vi "tes assemble (fuzzy).vi"() -> ()   [LabVIEW 2015]
uses:
  <vilib>/userdefined/High Color/IMAQdx.ctl
  <vilib>/Platform/TimedLoop/XDataNode/timing_clust.ctl
  <vilib>/Platform/TimedLoop/XDataNode/nitl_modes.ctl
  <vilib>/Platform/TimedLoop/XDataNode/wakeup.ctl
  <vilib>/FPGAPlugInAG/myRIO-1900/niLvFpga_Open_myRIO-1900.vi
  <vilib>/rvi/interface/common/dynamic/niFpgaDynamicAddResources.vi
  <vilib>/FPGAPlugInAG/Dynamic/niLvFpga_Run_Dynamic.vi
  <vilib>/Utility/error.llb/Error Cluster From Error Code.vi
  <vilib>/rvi/errors/niLvFpgaAdjustHostInterfaceError.vi
  <vilib>/FPGAPlugInAG/Dynamic/niLvFpga_Close_Dynamic.vi
  <vilib>/addons/control/pid/pid.llb/PID (DBL).vi
  <vilib>/addons/Fuzzy Logic/FL Fuzzy Controller (MIMO).vi
  <vilib>/Platform/TimedLoop/XDataNode/XDataNode.xnode
  <vilib>/rvi/interface/nirviOpenFPGA/nirviOpenFPGA.xnode
  TA/FPGA Bitfiles/FPGAv2_FPGATarget2_Assemble_19Xc0cZodWc.lvbitx
  Assemble.vi
  <vilib>/rvi/interface/nirviMethod/nirviMethod.xnode
  <vilib>/rvi/interface/nirviReadWriteControl/nirviReadWriteControl.xnode
  <vilib>/rvi/interface/nirviCloseFPGA/nirviCloseFPGA.xnode
  <vilib>/rvi/interface/Simulation/niFpgaSimulationCallBeginRW.vi
  <vilib>/Platform/TimedLoop/XDataNode/XDNodeRunTimeDep.lvlib
  <vilib>/vision/driver/NI_Vision_Acquisition_Software.lvlib
  <resource>/objmgr/imaqdx.rc
  <vilib>/addons/control/pid/NI_PID_pid.lvlib
  NiFpgaLv.dll
  <vilib>/addons/Fuzzy Logic/NI_Fuzzy_Logic_API.lvlib
panel:
  out "voltage":dbl
  out "var.RTH":dbl
  out "kec.kanan":dbl
  out "kec.kiri":dbl
  out "kecp.kanan":dbl
  out "kecp.kiri":dbl
  out "var.auto":dbl
  out "Return to Home":dbl
  out "s 4":dbl
  out "s 3":dbl
  out "s 2":dbl
  out "s1":dbl
  out "var. auto":dbl
  in  "Mode":bool
  in  "Run/Stop":bool
  in  "RTH":bool
  in  "Enc1 Reset":bool
  in  "Enc2 Reset":bool
  in  "Enc3 Reset":bool
  in  "Enc4 Reset":bool
  in  "Tfu":u32=10
  out "lf 2":dbl
  out "fr 2":i32
  out "fw 2":i32
  out "fl 2":i32
  out "br 2":dbl
  out "bw 2":i32
  out "rg 2":dbl
  out "st 2":i32
  in  "Trigger pulse interval  4":u32
  in  "Trigger pulse interval  3":u32
  in  "Trigger pulse interval  2":u32
  in  "Trigger pulse interval 1":u32
  out "Motor Response-Set Point vs. AcualSpeed":cluster{dbl, "Velocity (Counts/Interval)":i32}(graph)
  out "relay 4":bool
  out "relay 3":bool
  out "relay 2":bool
  out "relay1":bool
  out "bocor 2":bool
  out "Water_LVL2":u16
  out "Water_LVL1":u16
  out "bocor 1":bool
  out "Arus 4":dbl
  out "Arus 3":dbl
  out "Arus 2":dbl
  out "Arus1":dbl
  out "En 8":bool
  out "En 7":bool
  out "En 6":bool
  out "En 5":bool
  out "En 4":bool
  out "En 3":bool
  out "En 2":bool
  out "En 1":bool
  out "Rpm 4":i32
  out "Rpm 3":i32
  out "Rpm 2":i32
  out "Rpm 1":i32
  out "To":u32
  out "var. manual":dbl
  out "enc 4":i32
  out "enc 3":i32
  out "enc 2":i32
  out "enc 1":i32
  out "Time On4":dbl format="%.2f"
  out "Time On3":dbl format="%.2f"
  out "Time On2":dbl
  out "y position":dbl
  out "x position":dbl
  out "angle":dbl
  out "jarak tempuh":dbl
  out "Tf":u32
  out "Time On1":dbl
  out "distance4":sgl
  out "distance3":sgl
  out "distance2":sgl
  out "distance1":sgl
  out "Image":T1(plugin-control)
  in  "Image Type":T2 items=["Grayscale (U8)", "Grayscale (I16)", "Grayscale (SGL)", "Complex (CSG)", "RGB (U32)", "HSL (U32)", "RGB (U64)", "Grayscale (U16)"]
  in  "Border Size":i32=3
  in  "Session In":T3
  out "Channel 2":u32
  out "Channel 1":u32
  out "US 4":u32
  out "US3":u32
  out "US2":u32
  out "US1":u32
  out "STOP Indicator":bool
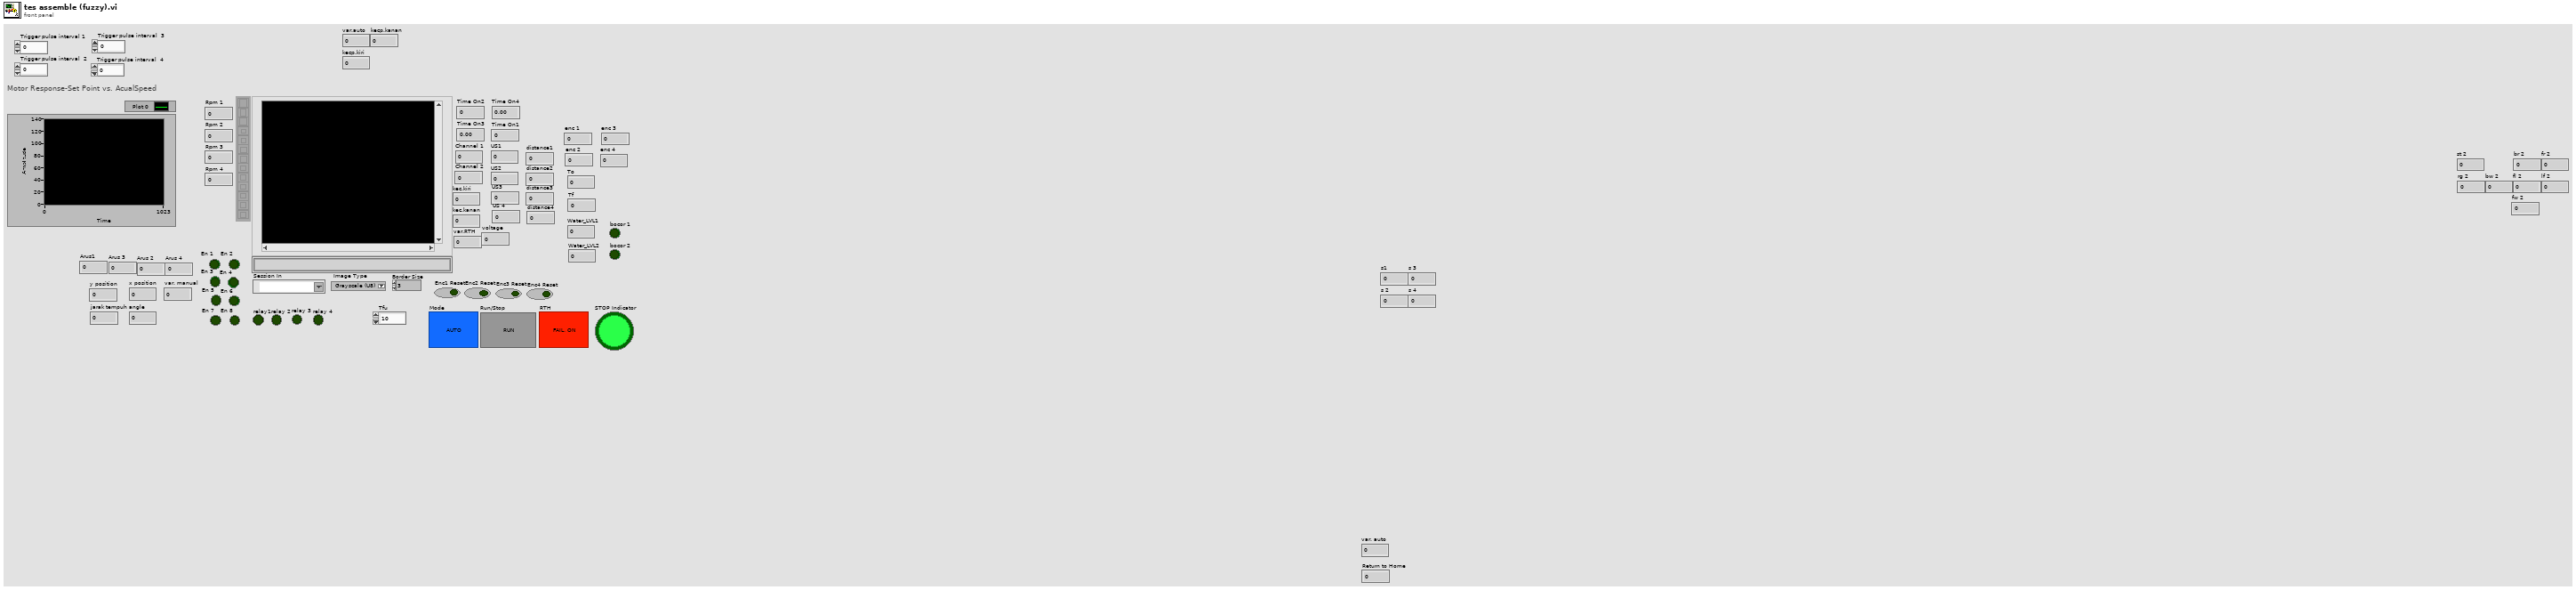
[diagram p1: front panel]
types:
  T1 = typedef "IMAQ Image.ctl" = refnum<image>
  T2 = typedef "Image Type" = u32
  T3 = typedef "IMAQdx.ctl" = refnum<k21>
  T4 = typedef "XDNodeRunTimeDep.lvlib/timing_clust.ctl" = cluster{"Expected End [f-1]":u64, "Actual End [f-1]":u64, "Finished Late? [f-1]":bool, "Expected End [i-1]":u64, "Actual End [i-1]":u64, "Finished Late? [i-1]":bool, "Expected Start [i]":u64, "Actual Start [i]":u64, "Expected Start [f]":u64, "Actual Start [f]":u64, "Source Name":string, "Structure Name":string, "Period":i64, "Deadline":i64, "Offset":i64, "Start":i64, "Priority":i32, "Timeout":i32, "Mode":T5, "Wakeup Reason":T6, "Error":errorcluster, "Source Type":string, "Secondary Source Type":string, "Global End Time":u64, "Global Start Time":u64, "Frame Duration":u64, "Iteration Duration":u64, "Assigned CPU":i32, "I/O Scan Engine Mode":u32}
  T5 = typedef "XDNodeRunTimeDep.lvlib/nitl_modes.ctl" = enum32{"No Change", "Process missed periods, maintain original phase", "Discard missed periods, maintain original phase", "Process missed periods, ignore original phase", "Discard missed periods, ignore original phase"}
  T6 = typedef "XDNodeRunTimeDep.lvlib/wakeup.ctl" = enum32{"Normal", "Aborted", "Asynchronous wakeup", "Timing source error", "Timed loop error", "Timeout"}
  T7 = cluster{"proportional gain (Kc)":dbl, "integral time (Ti, min)":dbl, "derivative time (Td, min)":dbl}
  T8 = typedef "NI_Fuzzy_Logic_API.lvlib/FL System.ctl" = cluster{"input variables":T9[], "output variables":T9[], "rules":T12[], "defuzzification method":T18, "description":string, "user MF interpolating polynomials":T19[]}
  T9 = typedef "NI_Fuzzy_Logic_API.lvlib/FL Variable.ctl" = cluster{"name":string, "range":dbl[], "MFs":T10[]}
  T10 = typedef "NI_Fuzzy_Logic_API.lvlib/FL Membership Function.ctl" = cluster{"name":string, "shape":T11, "points":dbl[], "color":u32, "user-defined shape index":i32}
  T11 = typedef "NI_Fuzzy_Logic_API.lvlib/FL Membership Function Shape.ctl" = u16
  T12 = typedef "NI_Fuzzy_Logic_API.lvlib/FL Rule.ctl" = cluster{"antecedents":T13[], "antecedent connective":T15, "consequents":T16[], "consequent implication":T17, "degree of support":dbl}
  T13 = typedef "NI_Fuzzy_Logic_API.lvlib/FL Antecedent.ctl" = cluster{"Var Index":i32, "MF Index":i32, "Cond":T14}
  T14 = typedef "NI_Fuzzy_Logic_API.lvlib/FL Modifier.ctl" = u16
  T15 = typedef "NI_Fuzzy_Logic_API.lvlib/FL Antecedent Connective.ctl" = u16
  T16 = typedef "NI_Fuzzy_Logic_API.lvlib/FL Consequent.ctl" = cluster{"Var Index":i32, "MF Index":i32, "Cond":T14}
  T17 = typedef "NI_Fuzzy_Logic_API.lvlib/FL Consequent Implication.ctl" = u16
  T18 = typedef "NI_Fuzzy_Logic_API.lvlib/FL Defuzzification.ctl" = u16
  T19 = typedef "NI_Fuzzy_Logic_API.lvlib/FL Interpolating polynomials.ctl" = cluster{"X":dbl[], "Y":dbl[], "Y(x) coeff":dbl[][], "X(y) coeff":dbl[][], "Area(y) coeff":dbl[][], "coa_x(y) coeff":dbl[][]}
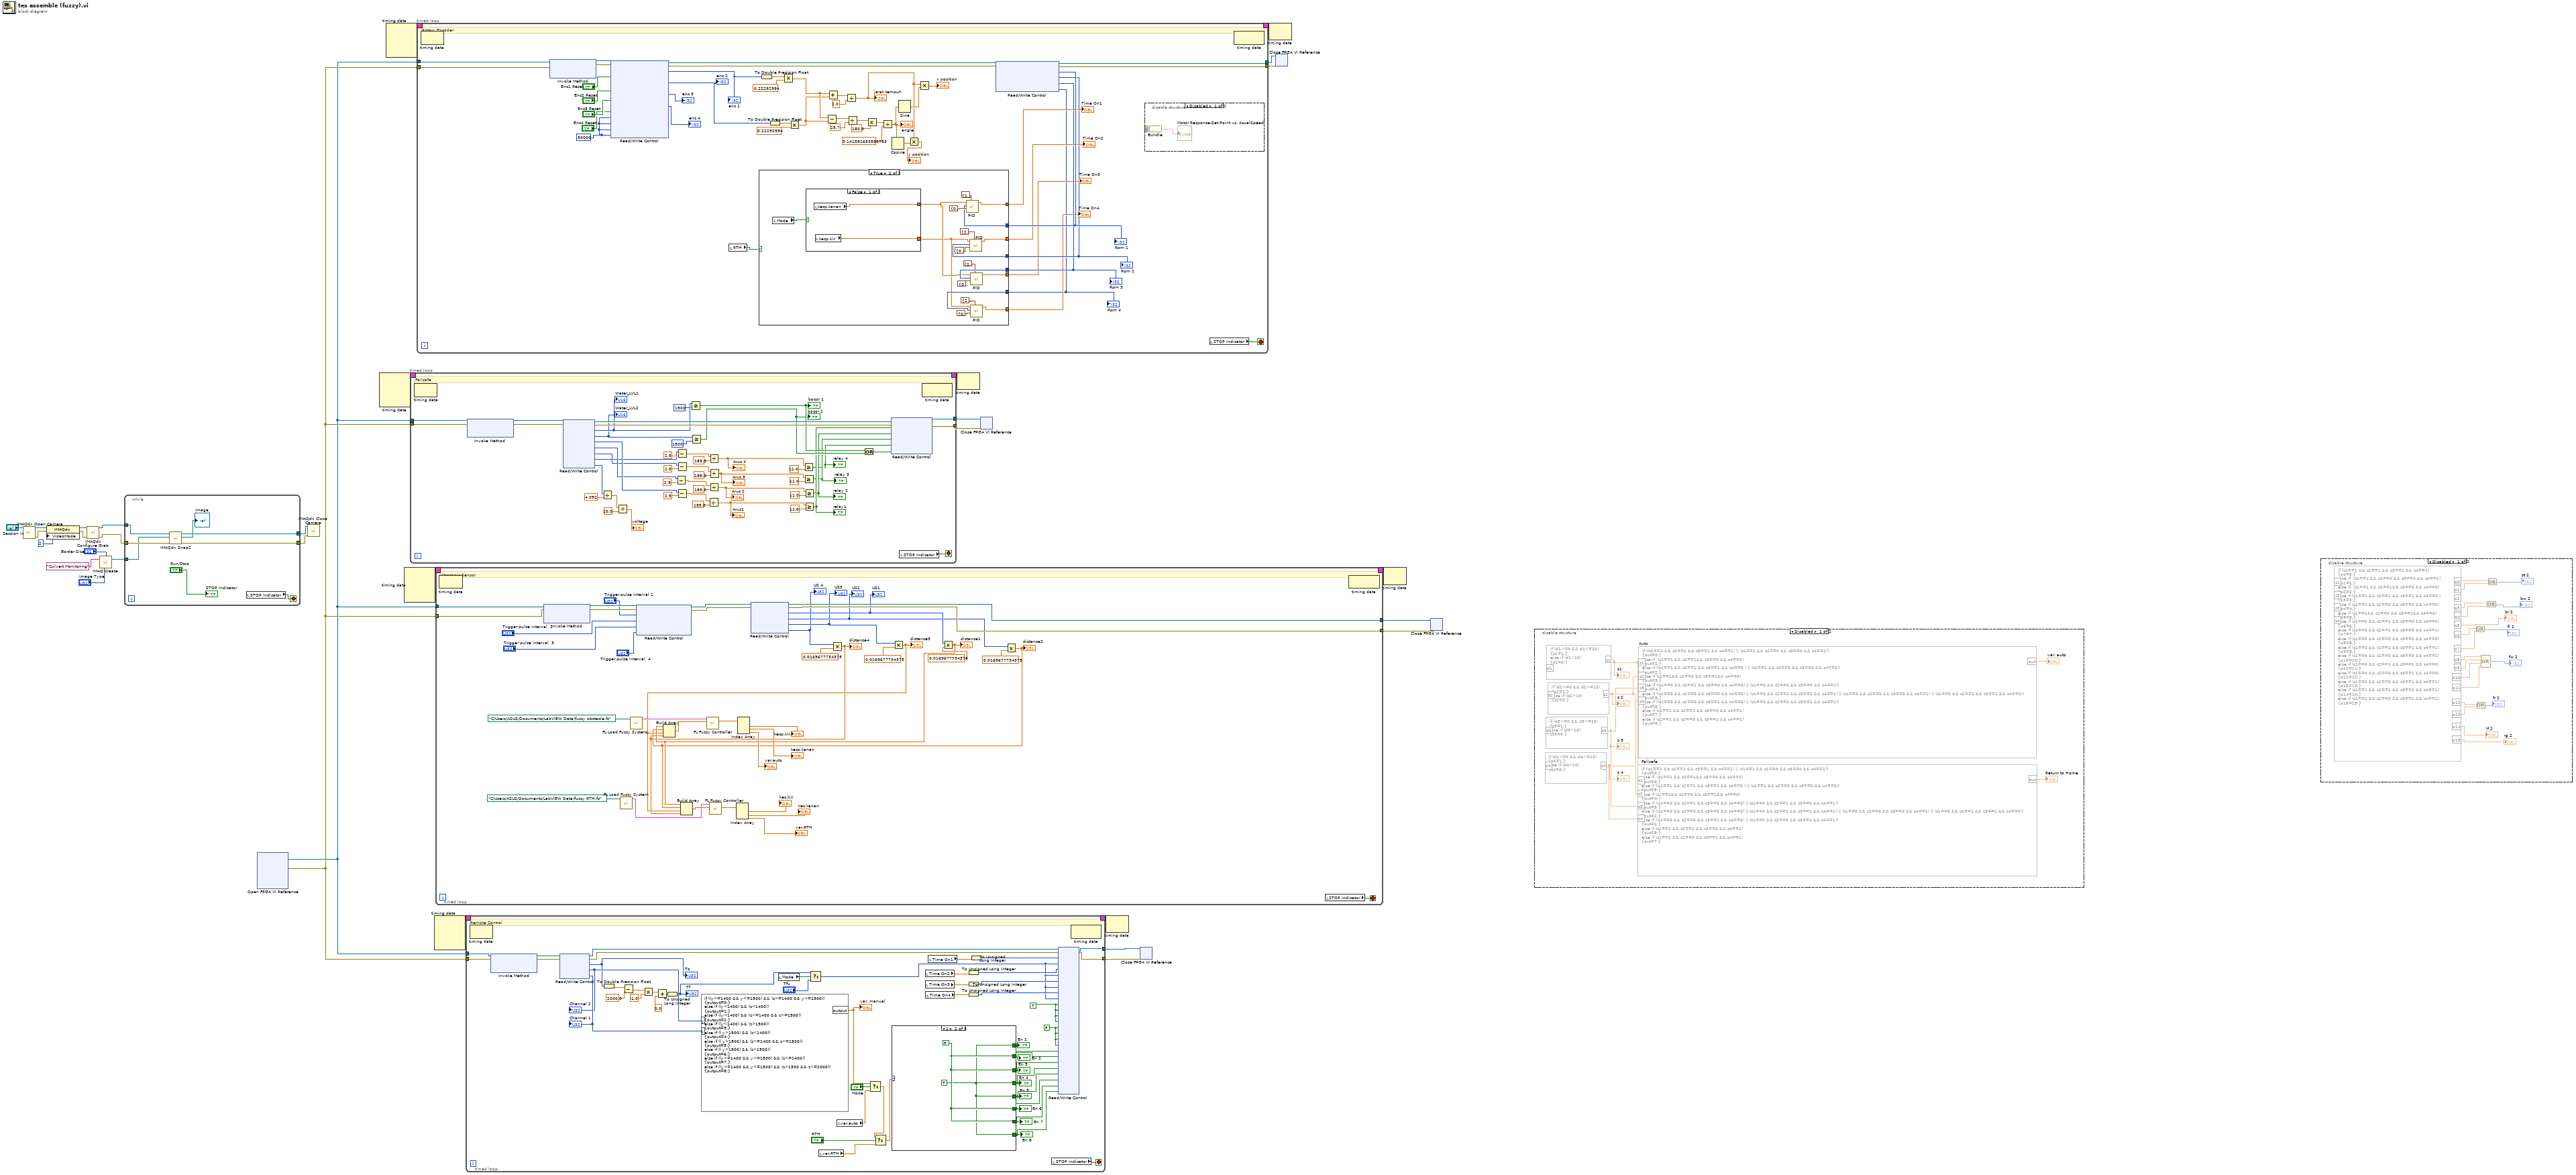
[diagram p0: block diagram]
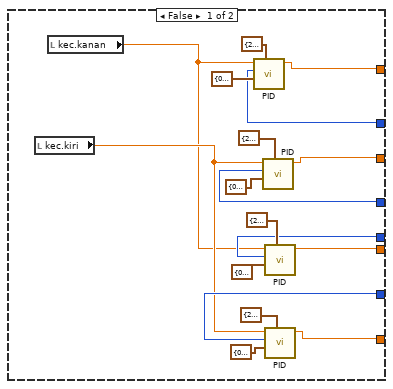
[diagram p4: hidden frame]
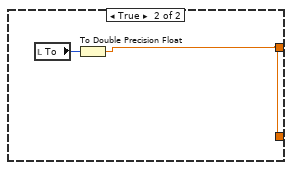
[diagram p5: hidden frame]
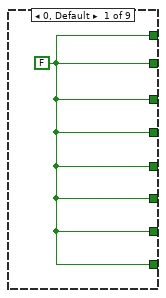
[diagram p7: hidden frame]
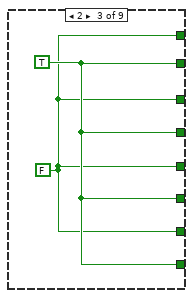
[diagram p8: hidden frame]
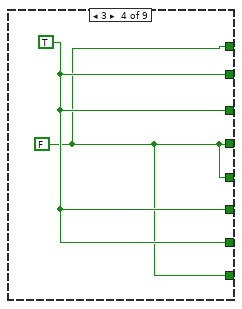
[diagram p9: hidden frame]
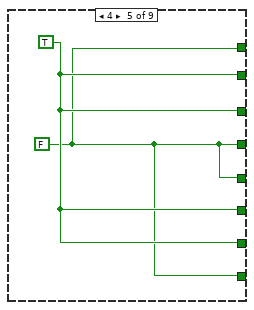
[diagram p10: hidden frame]
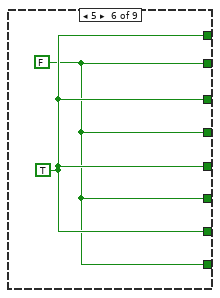
[diagram p11: hidden frame]
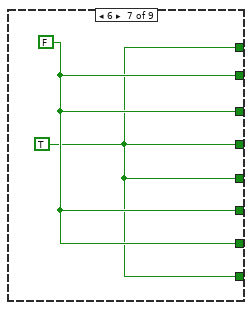
[diagram p12: hidden frame]
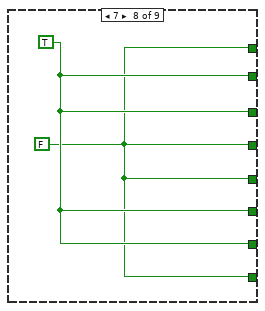
[diagram p13: hidden frame]
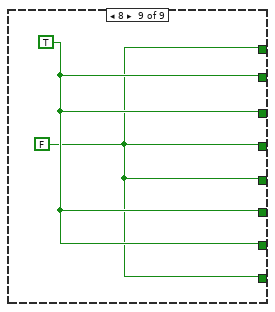
[diagram p14: hidden frame]
diagram:
  n1 = call <vilib>:"IMAQdx Open Camera.vi"("Session In"="Session In") -> ("error out"=w18:errorcluster, "Session Out"=w20:T3)  [unwired: 9 in]
  n2 = property class="IMAQdx"(reference=w20, error in=w18, "VideoMode"=u32 2) -> (reference out=w19:T3, error out=w17:errorcluster)
  n3 = call <vilib>:"IMAQdx Configure Grab.vi"("error in"=w17, "Session In"=w19) -> ("error out"=w14:errorcluster, "Session Out"=w15:T3)  [unwired: 8 in]
  n4 = call "IMAQ Create"("Border Size"="Border Size", "Image Name"="Culvert Monitoring", "Image Type"="Image Type") -> ("New Image"=w13:T1)  [unwired: 2 in, 1 out]
  n5 = while {
    tunnel: w15 -> [w35]
    tunnel: w14 -> [w37]
    tunnel: w13 -> [w36]
    tunnel: [w34] -> w12
    tunnel: [w33] -> w11
    stop <- w39 stop-if-true
    n6 = call <vilib>:"IMAQdx Snap2.vi"("error in"=w37, "Image In"=w36, "Session In"=w35) -> ("error out"=w33:errorcluster, "Image Out"=→"Image":T1, "Session Out"=w34:T3)  [unwired: 6 in]
    n7 = local read "STOP Indicator"() -> (w39:bool)
    "STOP Indicator" <- "Run/Stop"
  }
  n8 = xnode "Open FPGA VI Reference"() -> ("FPGA VI Reference Out"=w4:refnum<k20>, "error out"=w3:errorcluster)  [unwired: 2 in]
  n9 = call <vilib>:"IMAQdx Close Camera.vi"("error in"=w11, "Session In"=w12) -> ()  [unwired: 9 in, 1 out]
  n10 = node-c288() -> (w6:T4)  [unwired: 4 in]
  n11 = node-c288() -> (w10:T4)  [unwired: 4 in]
  n12 = node-c288() -> (w28:T4)  [unwired: 4 in]
  n13 = timed-loop {
    timing: w6 -> [_]
    timing-out: [_] -> w5
    tunnel: w4 -> [w89]
    tunnel: w3 -> [w88]
    tunnel: [w83] -> w2
    tunnel: [w82] -> w1
    stop <- w81 stop-if-true
    # "Failsafe"
    n14 = node-c288() -> ()  [unwired: 1 in, 1 out]
    n15 = xnode "Invoke Method"("FPGA VI Reference In"=w89, "error in"=w88) -> ("FPGA VI Reference Out"=w87:refnum<k20>, "error out"=w86:errorcluster)  [unwired: 1 in]
    n16 = xnode "Read/Write Control"("FPGA VI Reference In"=w87, "error in"=w86) -> ("FPGA VI Reference Out"=w85:refnum<k20>, "error out"=w84:errorcluster, "Water_LVL1"=w64:u16, "Water_LVL2"=w61:u16, "ACS712(1)"=w68:u16, "ACS712(2)"=w67:u16, "ACS712(3)"=w66:u16, "ACS712(4)"=w65:u16, "V sensor"=w44:u16)
    "Water_LVL1" <- w64
    "Water_LVL2" <- w61
    n17 = Divide(x=w44, y=4.092) -> (x/y=w43:dbl)
    n18 = Divide(x=w43, y=10.0) -> (x/y=→"voltage":dbl)
    n19 = Subtract(x=w67, y=2.5) -> (x-y=w71:dbl)
    n20 = Subtract(x=w65, y=2.5) -> (x-y=w75:dbl)
    n21 = Subtract(x=w66, y=2.5) -> (x-y=w73:dbl)
    n22 = Subtract(x=w68, y=2.5) -> (x-y=w69:dbl)
    n23 = Greater Or Equal?(x=w64, y=u16 1500) -> (x >= y?=w59:bool)
    "bocor 1" <- w59
    n24 = Greater Or Equal?(x=w61, y=u16 1500) -> (x >= y?=w58:bool)
    "bocor 2" <- w58
    n25 = Divide(x=w69, y=185.0) -> (x/y=w57:dbl)
    "Arus1" <- w57
    n26 = Divide(x=w75, y=185.0) -> (x/y=w49:dbl)
    "Arus 4" <- w49
    n27 = Divide(x=w71, y=185.0) -> (x/y=w53:dbl)
    "Arus 2" <- w53
    n28 = Divide(x=w73, y=185.0) -> (x/y=w51:dbl)
    "Arus 3" <- w51
    n29 = Greater Or Equal?(x=w49, y=11.0) -> (x >= y?=w46:bool)
    "relay 4" <- w46
    n30 = Greater Or Equal?(x=w51, y=11.0) -> (x >= y?=w47:bool)
    "relay 3" <- w47
    n31 = Greater Or Equal?(x=w53, y=11.0) -> (x >= y?=w48:bool)
    "relay 2" <- w48
    n32 = Greater Or Equal?(x=w57, y=11.0) -> (x >= y?=w55:bool)
    "relay1" <- w55
    n33 = Or(x=w59, y=w58) -> (x .or. y?=w60:bool)
    n34 = xnode "Read/Write Control"("FPGA VI Reference In"=w85, "error in"=w84, "Relay Motor 1"=w55, "Relay motor 2"=w48, "Relay motor 3"=w47, "Relay motor 4"=w46, "Relay kebocoran"=w60) -> ("FPGA VI Reference Out"=w83:refnum<k20>, "error out"=w82:errorcluster)
    n35 = local read "STOP Indicator"() -> (w81:bool)
    n36 = node-c288() -> ()  [unwired: 1 in, 1 out]
  }
  n37 = timed-loop {
    timing: w10 -> [_]
    timing-out: [_] -> w9
    tunnel: w4 -> [w136]
    tunnel: w3 -> [w135]
    tunnel: [w106] -> w8
    tunnel: [w105] -> w7
    stop <- w133 stop-if-true
    w102 = u32 50000 ("Velocity Interval (uSec) 4")
    # "Rotary Encoder"
    n38 = node-c288() -> ()  [unwired: 1 in, 1 out]
    n39 = xnode "Invoke Method"("FPGA VI Reference In"=w136, "error in"=w135) -> ("FPGA VI Reference Out"=w138:refnum<k20>, "error out"=w137:errorcluster)  [unwired: 1 in]
    n40 = xnode "Read/Write Control"("FPGA VI Reference In"=w138, "error in"=w137, "Position Reset"="Enc1 Reset", "Position Reset 2"="Enc2 Reset", "Position Reset 3"="Enc3 Reset", "Position Reset 4"="Enc4 Reset", "Velocity Interval (uSec)"=w102, "Velocity Interval (uSec) 2"=w102, "Velocity Interval (uSec) 3"=w102, "Velocity Interval (uSec) 4"=w102) -> ("FPGA VI Reference Out"=w104:refnum<k20>, "error out"=w103:errorcluster, "Position 1"=w107:i32, "Position 2"=w112:i32, "Position 3"=→"enc 3":i32, "Position 4"=→"enc 4":i32)
    "enc 1" <- w107
    "enc 2" <- w112
    n41 = local read "RTH"() -> (w92:bool)
    n42 = To Double Precision Float(number=w107) -> (double precision float=w132:dbl)
    n43 = To Double Precision Float(number=w112) -> (double precision float=w131:dbl)
    n44 = Multiply(x=w132, y=0.22292994) -> (x*y=w126:dbl)
    n45 = Multiply(x=w131, y=0.22292994) -> (x*y=w125:dbl)
    n46 = Subtract(x=w126, y=w125) -> (x-y=w124:dbl)
    n47 = Add(x=w126, y=w125) -> (x+y=w128:dbl)
    n48 = Divide(x=w128, y=2.0) -> (x/y=w115:dbl)
    "jarak tempuh" <- w115
    n49 = Divide(x=w124, y=25.7) -> (x/y=w122:dbl)
    n50 = Multiply(x=w122, y=180.0) -> (x*y=w120:dbl)
    n51 = Divide(x=w120, y=3.141592653589793) -> (x/y=w118:dbl)
    "angle" <- w118
    n52 = Cosine(x=w118) -> (cos(x)=w116:dbl)
    n53 = Sine(x=w118) -> (sin(x)=w117:dbl)
    n54 = Multiply(x=w115, y=w116) -> (x*y=→"y position":dbl)
    n55 = Multiply(x=w115, y=w117) -> (x*y=→"x position":dbl)
    n56 = xnode "Read/Write Control"("FPGA VI Reference In"=w104, "error in"=w103) -> ("FPGA VI Reference Out"=w106:refnum<k20>, "error out"=w105:errorcluster, "Velocity (Counts/Interval)"=w100:i32, "Velocity (Counts/Interval) 2"=w97:i32, "Velocity (Counts/Interval) 3"=w96:i32, "Velocity (Counts/Interval) 4"=w93:i32)
    "Rpm 1" <- w100
    "Rpm 2" <- w97
    "Rpm 3" <- w96
    "Rpm 4" <- w93
    n57 = case shown="True" w92 {
      tunnel: w100 -> [w147 w172]
      tunnel: [w148 w171] -> w99
      tunnel: [w146 w168] -> w98
      tunnel: w97 -> [w145 w167]
      tunnel: w96 -> [w144 w164]
      tunnel: [w143 w163] -> w95
      tunnel: [w141 w160] -> w94
      tunnel: w93 -> [w142 w159]
      frame False {
        n58 = local read "kec.kiri"() -> (w140:dbl)
        n59 = local read "kec.kanan"() -> (w139:dbl)
        n60 = call-poly <vilib>:"PID.vi"("output range"=cluster{"output high":dbl, "output low":dbl} {"output high"=2000.0, "output low"=0.0}, "PID gains"=T7 {"proportional gain (Kc)"=0.3, "integral time (Ti, min)"=0.75, "derivative time (Td, min)"=0.1875}, "process variable"=w147, "setpoint"=w139) -> ("output"=w148:dbl)  [unwired: 6 in, 1 out]
        n61 = call-poly <vilib>:"PID.vi"("output range"=cluster{"output high":dbl, "output low":dbl} {"output high"=2000.0, "output low"=0.0}, "PID gains"=T7 {"proportional gain (Kc)"=0.3, "integral time (Ti, min)"=0.75, "derivative time (Td, min)"=0.1875}, "process variable"=w145, "setpoint"=w140) -> ("output"=w146:dbl)  [unwired: 6 in, 1 out]
        n62 = call-poly <vilib>:"PID.vi"("output range"=cluster{"output high":dbl, "output low":dbl} {"output high"=2000.0, "output low"=0.0}, "PID gains"=T7 {"proportional gain (Kc)"=0.3, "integral time (Ti, min)"=0.75, "derivative time (Td, min)"=0.1875}, "process variable"=w144, "setpoint"=w139) -> ("output"=w143:dbl)  [unwired: 6 in, 1 out]
        n63 = call-poly <vilib>:"PID.vi"("output range"=cluster{"output high":dbl, "output low":dbl} {"output high"=2000.0, "output low"=0.0}, "PID gains"=T7 {"proportional gain (Kc)"=0.3, "integral time (Ti, min)"=0.75, "derivative time (Td, min)"=0.1875}, "process variable"=w142, "setpoint"=w140) -> ("output"=w141:dbl)  [unwired: 6 in, 1 out]
      }
      frame True {
        n64 = local read "Mode"() -> (w175:bool)
        n65 = case shown="False" w175 {
          tunnel: [w176 w178] -> w157
          tunnel: [w177 w178] -> w158
          frame False {
            n66 = local read "kecp.kanan"() -> (w177:dbl)
            n67 = local read "kecp.kiri"() -> (w176:dbl)
          }
          frame True {
            n68 = local read "To"() -> (w179:u32)
            n69 = To Double Precision Float(number=w179) -> (double precision float=w178:dbl)
          }
        }
        n70 = call-poly <vilib>:"PID.vi"("output range"=cluster{"output high":dbl, "output low":dbl} {"output high"=2000.0, "output low"=0.0}, "PID gains"=T7 {"proportional gain (Kc)"=0.3, "integral time (Ti, min)"=0.75, "derivative time (Td, min)"=0.1875}, "process variable"=w172, "setpoint"=w158) -> ("output"=w171:dbl)  [unwired: 6 in, 1 out]
        n71 = call-poly <vilib>:"PID.vi"("output range"=cluster{"output high":dbl, "output low":dbl} {"output high"=2000.0, "output low"=0.0}, "PID gains"=T7 {"proportional gain (Kc)"=0.3, "integral time (Ti, min)"=0.75, "derivative time (Td, min)"=0.1875}, "process variable"=w167, "setpoint"=w157) -> ("output"=w168:dbl)  [unwired: 6 in, 1 out]
        n72 = call-poly <vilib>:"PID.vi"("output range"=cluster{"output high":dbl, "output low":dbl} {"output high"=2000.0, "output low"=0.0}, "PID gains"=T7 {"proportional gain (Kc)"=0.3, "integral time (Ti, min)"=0.75, "derivative time (Td, min)"=0.1875}, "process variable"=w164, "setpoint"=w158) -> ("output"=w163:dbl)  [unwired: 6 in, 1 out]
        n73 = call-poly <vilib>:"PID.vi"("output range"=cluster{"output high":dbl, "output low":dbl} {"output high"=2000.0, "output low"=0.0}, "PID gains"=T7 {"proportional gain (Kc)"=0.3, "integral time (Ti, min)"=0.75, "derivative time (Td, min)"=0.1875}, "process variable"=w159, "setpoint"=w157) -> ("output"=w160:dbl)  [unwired: 6 in, 1 out]
      }
    }
    "Time On1" <- w99
    "Time On2" <- w98
    "Time On3" <- w95
    "Time On4" <- w94
    n74 = disable-structure shown="Disabled" {
      disable-tunnel: _ -> [w182 _]
      disable-tunnel: _ -> [w180 _]
      frame Disabled {
        n75 = Bundle(w180, w182) -> (→"Motor Response-Set Point vs. AcualSpeed":cluster{void, void})  [unwired: 1 in]
      }
      frame Enabled {
      }
    }
    n76 = local read "STOP Indicator"() -> (w133:bool)
    n77 = node-c288() -> ()  [unwired: 1 in, 1 out]
  }
  n78 = node-c288() -> (w30:T4)  [unwired: 4 in]
  n79 = timed-loop {
    timing: w28 -> [_]
    timing-out: [_] -> w27
    tunnel: [w220] -> w26
    tunnel: [w219] -> w25
    tunnel: w4 -> [w218]
    tunnel: w3 -> [w217]
    stop <- w223 stop-if-true
    # "Ultrasonic Sensor"
    n80 = node-c288() -> ()  [unwired: 1 in, 1 out]
    n81 = xnode "Invoke Method"("FPGA VI Reference In"=w218, "error in"=w217) -> ("FPGA VI Reference Out"=w216:refnum<k20>, "error out"=w215:errorcluster)  [unwired: 1 in]
    n82 = call <vilib>:"FL Load Fuzzy System.vi"("file path"=path "C:/Users/ASUS/Documents/LabVIEW Data/fuzzy RTH.fs") -> ("fuzzy system out"=w190:T8)  [unwired: 1 in, 9 out]
    n83 = call <vilib>:"FL Load Fuzzy System.vi"("file path"=path "C:/Users/ASUS/Documents/LabVIEW Data/fuzzy obstacle.fs") -> ("fuzzy system out"=w203:T8)  [unwired: 1 in, 9 out]
    n84 = xnode "Read/Write Control"("FPGA VI Reference In"=w216, "error in"=w215, "Trigger pulse interval 1"="Trigger pulse interval 1", "Trigger pulse interva 2"="Trigger pulse interval  2", "Trigger pulse interval 3"="Trigger pulse interval  3", "Trigger pulse interval 4"="Trigger pulse interval  4") -> ("FPGA VI Reference Out"=w222:refnum<k20>, "error out"=w221:errorcluster)
    n85 = xnode "Read/Write Control"("FPGA VI Reference In"=w222, "error in"=w221) -> ("FPGA VI Reference Out"=w220:refnum<k20>, "error out"=w219:errorcluster, "time of flight 1"=w214:u32, "time of flight 2"=w213:u32, "time of flight 3"=w210:u32, "time of flight 4"=w208:u32)
    "US1" <- w214
    "US2" <- w213
    "US3" <- w210
    "US 4" <- w208
    n86 = Multiply(x=w208, y=sgl 0.016967773) -> (x*y=w192:sgl)
    "distance4" <- w192
    n87 = Multiply(x=w210, y=sgl 0.016967773) -> (x*y=w193:sgl)
    "distance3" <- w193
    n88 = Multiply(x=w214, y=sgl 0.016967773) -> (x*y=w195:sgl)
    "distance1" <- w195
    n89 = Multiply(x=w213, y=sgl 0.016967773) -> (x*y=w194:sgl)
    "distance2" <- w194
    n90 = Build Array(w195, w194, w193, w192) -> (w200:sgl[])
    n91 = Build Array(w195, w194, w193, w192) -> (w191:sgl[])
    n92 = call-poly <vilib>:"FL Fuzzy Controller.vi"("input values"=w200, "fuzzy system in"=w203) -> ("output values"=w199:dbl[])  [unwired: 1 in, 8 out]
    n93 = call-poly <vilib>:"FL Fuzzy Controller.vi"("input values"=w191, "fuzzy system in"=w190) -> ("output values"=w188:dbl[])  [unwired: 1 in, 8 out]
    n94 = Index Array(array=w188) -> (element #1=→"kec.kiri":dbl, element #2=→"kec.kanan":dbl, element #3=→"var.RTH":dbl)  [unwired: 3 in]
    n95 = Index Array(array=w199) -> (element #1=→"kecp.kiri":dbl, element #2=→"kecp.kanan":dbl, element #3=→"var.auto":dbl)  [unwired: 3 in]
    n96 = local read "STOP Indicator"() -> (w223:bool)
    n97 = node-c288() -> ()  [unwired: 1 in, 1 out]
  }
  n98 = timed-loop {
    tunnel: [w258] -> w32
    tunnel: [w256] -> w31
    timing: w30 -> [_]
    timing-out: [_] -> w29
    tunnel: w4 -> [w272]
    tunnel: w3 -> [w271]
    stop <- w273 stop-if-true
    w226 = TRUE ("E2O")
    w254 = FALSE ("EI1")
    # "Remote Control"
    n99 = node-c288() -> ()  [unwired: 1 in, 1 out]
    n100 = xnode "Invoke Method"("FPGA VI Reference In"=w272, "error in"=w271) -> ("FPGA VI Reference Out"=w270:refnum<k20>, "error out"=w269:errorcluster)  [unwired: 1 in]
    n101 = xnode "Read/Write Control"("FPGA VI Reference In"=w270, "error in"=w269) -> ("FPGA VI Reference Out"=w257:refnum<k20>, "error out"=w255:errorcluster, "Channel 3"=w236:u32, "Channel) 2"=w267:u32, "Channel 1"=w268:u32)
    "Channel 1" <- w268
    "Channel 2" <- w267
    "To" <- w236
    n102 = To Double Precision Float(number=w236) -> (double precision float=w260:dbl)
    n103 = Subtract(x=w260, y=sgl 2000.0) -> (x-y=w266:dbl)
    n104 = Multiply(x=w266, y=sgl -1.0) -> (x*y=w265:dbl)
    n105 = Add(x=w265, y=sgl 0.0 ("-y")) -> (x+y=w264:dbl)
    n106 = To Unsigned Long Integer(number=w264) -> (unsigned 32bit integer=w234:u32)
    "Tf" <- w234
    n107 = formula code="if ((y>=1400 && y<=1500) && (z>=1400 && y<=1500))\n{output=0;} \nelse if ((y<1400) && (z<1400))\n{output=1;}\nelse if ((y<1400) && (z>=1400 && z<=1500))\n{output=2;}\nelse if ((y<1400) && (z>1500))\n{output=3;}\nelse if (( y>1500) && (z<1400))\n{output=4;}\nelse if (( y>1500) && (z>=1400 && z<=1500))\n{output=5;}\nelse if (( y>1500) && (z>1500))\n{output=6;}\nelse if ((y>=1400 && y<=1500) && (z<=1400))\n{output=7;}\nelse if ((y>=1400 && y<=1500) && (z>1500 && z<=2000))\n{output=8;}"("y"=w267, "z"=w268) -> ("output"=w238:dbl)
    "var. manual" <- w238
    n108 = local read "Mode"() -> (w232:bool)
    n109 = Select(t=w234, s=w232, f="Tfu") -> (s? t:f=w231:u32)
    n110 = local read "var.RTH"() -> (w228:dbl)
    n111 = local read "var.auto"() -> (w237:dbl)
    n112 = Select(t=w238, s="Mode", f=w237) -> (s? t:f=w230:dbl)
    n113 = Select(t=w230, s="RTH", f=w228) -> (s? t:f=w229:dbl)
    n114 = case shown="1" w229 {
      tunnel: [w274 w275 w277 w279 w281 w284 w285 w287 w289] -> w252
      tunnel: [w274 w276 w278 w280 w282 w283 w286 w288 w290] -> w251
      tunnel: [w274 w276 w277 w280 w282 w284 w286 w288 w290] -> w250
      tunnel: [w274 w275 w278 w279 w281 w283 w285 w287 w289] -> w249
      tunnel: [w274 w275 w277 w279 w281 w284 w285 w287 w289] -> w248
      tunnel: [w274 w276 w278 w280 w282 w283 w286 w288 w290] -> w247
      tunnel: [w274 w276 w277 w280 w282 w284 w286 w288 w290] -> w246
      tunnel: [w274 w275 w278 w279 w281 w283 w285 w287 w289] -> w245
      frame 0, Default {
        w274 = FALSE ("En")
      }
      frame 1 {
        w275 = TRUE ("En")
        w276 = FALSE ("En")
      }
      frame 2 {
        w277 = FALSE ("En")
        w278 = TRUE ("En")
      }
      frame 3 {
        w279 = FALSE ("En")
        w280 = TRUE ("En")
      }
      frame 4 {
        w281 = FALSE ("En")
        w282 = TRUE ("En")
      }
      frame 5 {
        w284 = TRUE ("En")
        w283 = FALSE ("En")
      }
      frame 6 {
        w285 = TRUE ("En")
        w286 = FALSE ("En")
      }
      frame 7 {
        w287 = FALSE ("En")
        w288 = TRUE ("En")
      }
      frame 8 {
        w289 = FALSE ("En")
        w290 = TRUE ("En")
      }
    }
    "En 1" <- w252
    "En 2" <- w251
    "En 3" <- w250
    "En 4" <- w249
    "En 5" <- w248
    "En 6" <- w247
    "En 7" <- w246
    "En 8" <- w245
    n115 = local read "Time On2"() -> (w244:dbl)
    n116 = local read "Time On3"() -> (w243:dbl)
    n117 = local read "Time On4"() -> (w242:dbl)
    n118 = local read "Time On1"() -> (w259:dbl)
    n119 = To Unsigned Long Integer(number=w244) -> (unsigned 32bit integer=w241:u32)
    n120 = To Unsigned Long Integer(number=w243) -> (unsigned 32bit integer=w240:u32)
    n121 = To Unsigned Long Integer(number=w242) -> (unsigned 32bit integer=w239:u32)
    n122 = To Unsigned Long Integer(number=w259) -> (unsigned 32bit integer=w253:u32)
    n123 = local read "STOP Indicator"() -> (w273:bool)
    n124 = xnode "Read/Write Control"("FPGA VI Reference In"=w257, "error in"=w255, "ton"=w253, "tof"=w231, "ton 2"=w241, "tof 2"=w231, "ton 3"=w240, "tof 3"=w231, "ton 4"=w239, "tof 4"=w231, "E1O"=w226, "E2O"=w226, "E3O"=w226, "E4O"=w226, "EI1"=w254, "EI2"=w254, "EI3"=w254, "EI4"=w254, "En1"=w252, "En2"=w251, "En3"=w250, "En4"=w249, "En5"=w248, "En6"=w247, "En7"=w246, "En8"=w245) -> ("FPGA VI Reference Out"=w258:refnum<k20>, "error out"=w256:errorcluster)
    n125 = node-c288() -> ()  [unwired: 1 in, 1 out]
  }
  n126 = node-c288(w5) -> ()  [unwired: 1 out]
  n127 = xnode "Close FPGA VI Reference"("FPGA VI Reference In"=w2, "error in"=w1) -> ()  [unwired: 1 out]
  n128 = node-c288(w29) -> ()  [unwired: 1 out]
  n129 = xnode "Close FPGA VI Reference"("FPGA VI Reference In"=w32, "error in"=w31) -> ()  [unwired: 1 out]
  n130 = node-c288(w9) -> ()  [unwired: 1 out]
  n131 = xnode "Close FPGA VI Reference"("FPGA VI Reference In"=w8, "error in"=w7) -> ()  [unwired: 1 out]
  n132 = node-c288(w27) -> ()  [unwired: 1 out]
  n133 = xnode "Close FPGA VI Reference"("FPGA VI Reference In"=w26, "error in"=w25) -> ()  [unwired: 1 out]
  n134 = disable-structure shown="Disabled" {
    frame Disabled {
      n135 = formula code="if (d4>=0 && d4<=10)\n{s4=1;}\nelse if (d4>10)\n{s4=0;}"() -> ("s4"=w294:dbl)  [unwired: 1 in]
      "s 4" <- w294
      n136 = formula code="if (d3>=0 && d3<=10)\n{s3=1;}\nelse if (d3>10)\n{s3=0;}"() -> ("s3"=w295:dbl)  [unwired: 1 in]
      "s 3" <- w295
      n137 = formula code="if (d1>=0 && d1<=10)\n{s1=1;}\nelse if (d1>10)\n{s1=0;}"() -> ("s1"=w297:dbl)  [unwired: 1 in]
      "s1" <- w297
      n138 = formula code="if (d2>=0 && d2<=10)\n{s2=1;}\nelse if (d2>10)\n{s2=0;}"() -> ("s2"=w296:dbl)  [unwired: 1 in]
      "s 2" <- w296
      n139 = formula code="if ((c1==1 && c2==1 && c3==1 && c4==1) || (c1==1 && c2==0 && c3==0 && c4==1))\n{out=0;} \nelse if  (c1==1 && c2==1&& c3==0 && c4==0)\n{out=6;}\nelse if ((c1==1 && c2==1 && c3==1 && c4==0 ) || (c1==1 && c2==0 && c3==0 && c4==0))\n{out=5;}\nelse if (c1==1&& c2==0 && c3==1&& c4==0)\n{out=4;}\nelse if ((c1==0 && c2==1 && c3==0 && c4==0) || (c1==0 && c2==1 && c3==0 && c4==1))\n{out=3;}\nelse if ((c1==0 && c2==0 && c3==0 && c4==0) || (c1==0 && c2==1 && c3==1 && c4==1) || (c1==0 && c2==0 && c3==0 && c4==1) || (c1==0 && c2==1 && c3==1 && c4==0))\n{out=2;}\nelse if ((c1==0 && c2==0 && c3==1 && c4==0) || (c1==0 && c2==0 && c3==1 && c4==1))\n{out=1;}\nelse if (c1==1 && c2==1 && c3==0 && c4==1)\n{out=8;}\nelse if (c1==1 && c2==0 && c3==1 && c4==1)\n{out=7;}" "Failsafe"("c1"=w297, "c2"=w296, "c3"=w295, "c4"=w294) -> ("out"=→"Return to Home":dbl)
      n140 = formula code="if ((c1==1 && c2==1 && c3==1 && c4==1) || (c1==1 && c2==0 && c3==0 && c4==1))\n{out=0;} \nelse if  (c1==1 && c2==1&& c3==0 && c4==0)\n{out=1;}\nelse if ((c1==1 && c2==1 && c3==1 && c4==0 ) || (c1==1 && c2==0 && c3==0 && c4==0))\n{out=2;}\nelse if (c1==1&& c2==0 && c3==1&& c4==0)\n{out=3;}\nelse if ((c1==0 && c2==1 && c3==0 && c4==0) || (c1==0 && c2==1 && c3==0 && c4==1))\n{out=4;}\nelse if ((c1==0 && c2==0 && c3==0 && c4==0) || (c1==0 && c2==1 && c3==1 && c4==1) || (c1==0 && c2==0 && c3==0 && c4==1) || (c1==0 && c2==1 && c3==1 && c4==0))\n{out=5;}\nelse if ((c1==0 && c2==0 && c3==1 && c4==0) || (c1==0 && c2==0 && c3==1 && c4==1))\n{out=6;}\nelse if (c1==1 && c2==1 && c3==0 && c4==1)\n{out=7;}\nelse if (c1==1 && c2==0 && c3==1 && c4==1)\n{out=8;}" "Auto"("c1"=w297, "c2"=w296, "c3"=w295, "c4"=w294) -> ("out"=→"var. auto":dbl)
    }
    frame Enabled {
    }
  }
  n141 = disable-structure shown="Disabled" {
    frame Disabled {
      n142 = formula code="if (c1==1 && c2==1 && c3==1 && c4==1)\n{o0=0;} \nelse if  (c1==1 && c2==0 && c3==0 && c4==1)\n{o1=1;} \nelse if  (c1==1 && c2==1&& c3==0 && c4==0)\n{o2=2;}\nelse if (c1==1 && c2==1 && c3==1 && c4==0 ) \n{o3=3;}\nelse if (c1==1 && c2==0 && c3==0 && c4==0)\n{o4=4;}\nelse if (c1==1&& c2==0 && c3==1&& c4==0)\n{o5=5;}\nelse if (c1==0 && c2==1 && c3==0 && c4==0) \n{o6=6;}\nelse if (c1==0 && c2==1 && c3==0 && c4==1)\n{o7=7;}\nelse if (c1==0 && c2==0 && c3==0 && c4==0) \n{o8=8;}\nelse if (c1==0 && c2==1 && c3==1 && c4==1) \n{o9=9;}\nelse if (c1==0 && c2==0 && c3==0 && c4==1) \n{o10=10;}\nelse if (c1==0 && c2==1 && c3==1 && c4==0)\n{o11=11;}\nelse if (c1==0 && c2==0 && c3==1 && c4==0)\n{o12=12;}\nelse if (c1==0 && c2==0 && c3==1 && c4==1)\n{o13=13;}\nelse if (c1==1 && c2==1 && c3==0 && c4==1)\n{o14=14;}\nelse if (c1==1 && c2==0 && c3==1 && c4==1)\n{o15=15;}"() -> ("c3"=w300:dbl, "o0"=w320:dbl, "o1"=w319:dbl, "o2"=w318:dbl, "o3"=w317:dbl, "o4"=w316:dbl, "o5"=→"br 2":dbl, "o6"=w313:dbl, "o7"=w312:dbl, "o8"=w310:dbl, "o9"=w309:dbl, "o10"=w308:dbl, "o11"=w307:dbl, "o12"=w305:dbl, "o13"=w304:dbl, "o14"=→"lf 2":dbl, "o15"=→"rg 2":dbl)  [unwired: 3 in]
      n143 = Or(x=w313, y=w312) -> (x .or. y?=→"fl 2":i32)
      n144 = Or(x=w305, y=w304) -> (x .or. y?=→"fr 2":i32)
      n145 = Compound Arithmetic op=OR(w310, w309, w308, w307) -> (→"fw 2":i32)
      n146 = Or(x=w317, y=w316) -> (x .or. y?=→"bw 2":i32)
      n147 = Or(x=w320, y=w319) -> (x .or. y?=→"st 2":i32)
    }
    frame Enabled {
    }
  }
